vi "Actor Core.vi"(8 "error in":errorcluster, 11 "TestActor in":refnum<class "TestActor.lvclass">) -> (0 "error out":errorcluster, 3 "Actor out":refnum<class "Actor.lvclass">)   [LabVIEW 2015, in "TestActor.lvlib" / "TestActor.lvclass"]
doc: "(<B>Filename</B>: Actor Framework.lvlib:Actor.lvclass:Actor Core.vi)\n\nReceives messages to the actor, reacts to them, and initiates any error handling that may shut the actor down.\n\nDescendant classes may override this VI to append parallel tasks for the actor to complete while it handles messages. Overrides use the Call Parent Method node."
uses:
  TestActor.lvclass
  <vilib>/ActorFramework/Actor/Actor.lvclass
  TestActor.lvclass/TestActor.ctl
  <vilib>/ActorFramework/Actor/Actor.lvclass/Actor.ctl
  <vilib>/ActorFramework/Message Enqueuer/Message Enqueuer.lvclass/Message Enqueuer.ctl
  <vilib>/ActorFramework/Message Enqueuer/Init from Existing Queue.vi
  <vilib>/ActorFramework/Message Enqueuer/Enqueue.vi
  <vilib>/ActorFramework/Message Priority Queue/Priority Enqueue.vi
  <vilib>/ActorFramework/Stop Msg/Stop Msg.lvclass
  <vilib>/ActorFramework/Message Enqueuer/Message Enqueuer.lvclass
  CSPP_Core/Actors/CS++BaseActor/CS++BaseActor.lvclass
panel:
  out "Number":dbl
  in  "Stop Button":bool
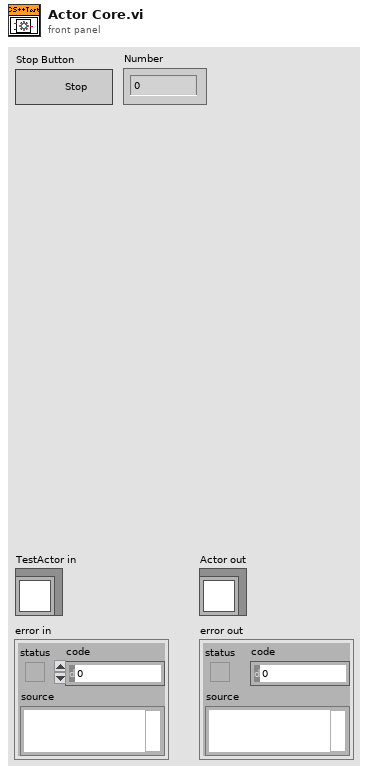
[diagram p1: front panel]
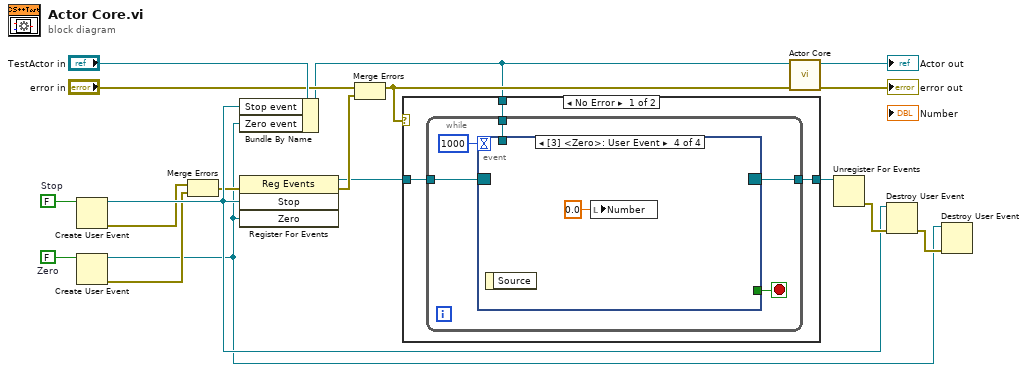
[diagram p0: block diagram]
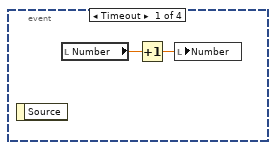
[diagram p2: hidden frame]
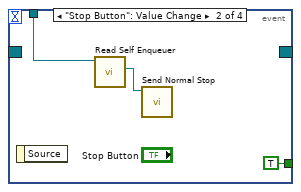
[diagram p3: hidden frame]
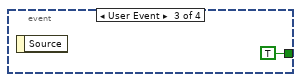
[diagram p4: hidden frame]
diagram:
  w6 = FALSE  # Zero
  w15 = FALSE  # Stop
  n1 = Create User Event(user event datatype=w15) -> (user event=w7:refnum<user-event>, error out=w5:errorcluster)  [unwired: 1 in]
  n2 = Create User Event(user event datatype=w6) -> (user event=w1:refnum<user-event>, error out=w3:errorcluster)  [unwired: 1 in]
  n3 = Merge Errors(w5, w3) -> (w4:errorcluster)
  n4 = Bundle By Name(cluster="TestActor in", "Stop event"=w7, "Zero event"=w1) -> (w8:refnum<class "TestActor.lvclass">)
  n5 = register-events(error in=w4, w7, w1) -> (reference out=w11:refnum<event-registration>, error out=w12:errorcluster)  [unwired: 1 in]
  n6 = Merge Errors("error in", w12) -> (w13:errorcluster)
  n7 = case shown="No Error" w13 {
    tunnel: w8 -> [w21 _]
    tunnel: w11 -> [w20 w34]
    tunnel: [w19 w34] -> w10
    frame No Error {
      n8 = while {
        tunnel: w21 -> [w24]
        tunnel: w20 -> [w23]
        tunnel: [w22] -> w19
        stop <- w25 stop-if-true
        n9 = event shown="[3] <Zero>: User Event" {
          selector: w23 -> [_ _ _ _]
          dyn-events: [_ _ _ _] -> w22
          timeout: 1000 -> [_ _ _ _]
          tunnel: [_ TRUE TRUE _] -> w25
          tunnel: w24 -> [_ w29 _ _]
          event Timeout {
            n10 = event-data() -> ()  [unwired: 1 in, 1 out]
            n11 = local read "Number"() -> (w28:dbl)
            n12 = Increment(x=w28) -> (x+1=w27:dbl)
            n13 = local write "Number"(w27) -> ()
          }
          event "Stop Button": Value Change {
            n14 = event-data() -> ()  [unwired: 1 in, 1 out]
            n15 = call <vilib>:"Read Self Enqueuer.vi"("Actor"=w29) -> ("Self Enqueuer"=w30:refnum<class "Message Enqueuer.lvclass">)  [unwired: 10 in]
            n16 = call <vilib>:"Send Normal Stop.vi"("Message Enqueuer"=w30) -> ()  [unwired: 10 in, 1 out]
          }
          event User Event {
            n17 = event-data() -> ()  [unwired: 1 in, 1 out]
          }
          event User Event {
            n18 = event-data() -> ()  [unwired: 1 in, 1 out]
            n19 = local write "Number"(0.0 ("Number")) -> ()
          }
        }
      }
    }
    frame Error {
    }
  }
  n20 = call-parent "Actor Core.vi"("error in"=w13, "CS++BaseActor in"=w8) -> ("error out"=→"error out":errorcluster, "Actor out"=→"Actor out":refnum<class "Actor.lvclass">)  [unwired: 8 in]
  n21 = Unregister For Events(event registration refnum=w10) -> (error out=w9:errorcluster)  [unwired: 1 in]
  n22 = Destroy User Event(user event=w7, error in=w9) -> (error out=w2:errorcluster)
  n23 = Destroy User Event(user event=w1, error in=w2) -> ()  [unwired: 1 out]
